vi "Find Steps to Reach End.vi"(0 "Start position":string, 1 "Map":map{string, cluster{string, string}}(c390), 3 "End condition":string, 4 "Instructions":string, 5 "Reach End this many times (1)":u64=1) -> (7 "Steps to reach last end":u64, 8 "End Reached at these steps":u64[](array[numeric]))   [LabVIEW 2020, in "AoC 2023.lvlib"]
uses:
  AoC 2023.lvlib
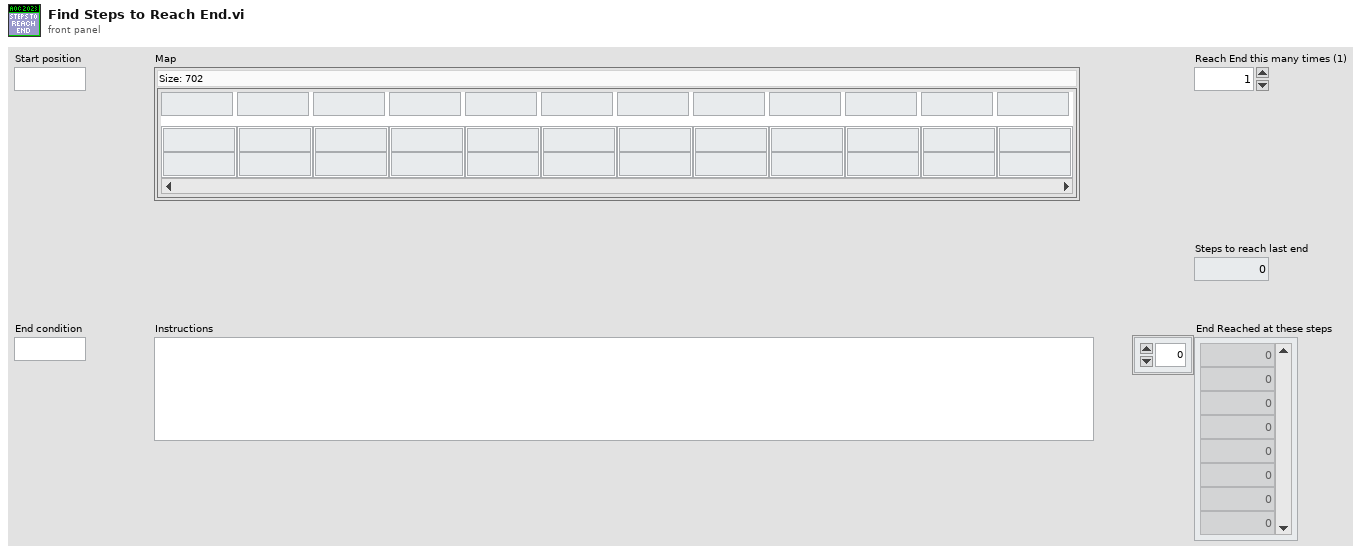
[diagram p1: front panel]
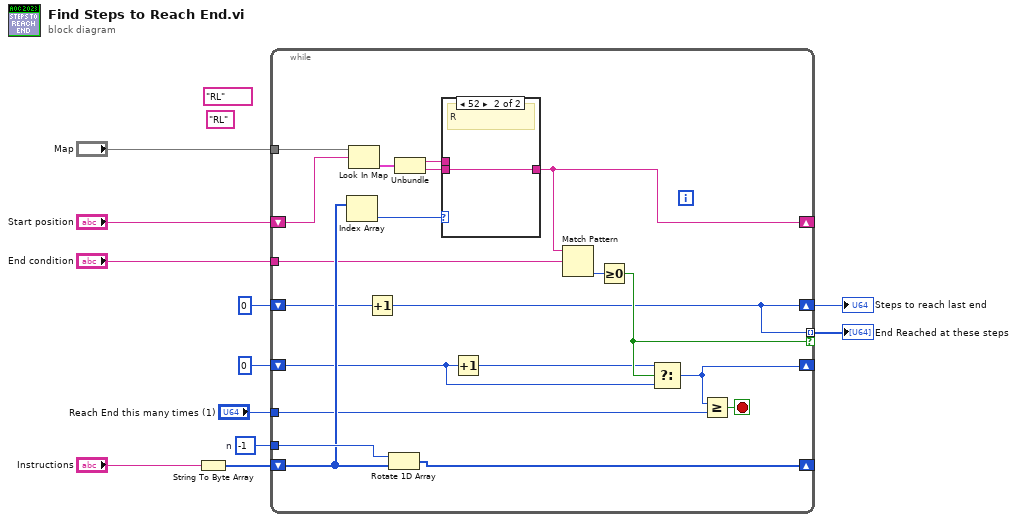
[diagram p0: block diagram]
diagram:
  w7 = -1  # n
  (unwired) "RL"
  (unwired) "RL"
  n1 = String To Byte Array(string="Instructions") -> (unsigned byte array=w6:u8[])
  n2 = while {
    tunnel: "Map" -> [w28]
    shift-right: [w31] -> _
    shift-left: w6 -> [w29]
    shift-right: [w25] -> _
    shift-left: "Start position" -> [w27]
    tunnel: w7 -> [w30]
    shift-right: [w21] -> w9
    shift-left: u64 0 -> [w24]
    tunnel: "End condition" -> [w23]
    tunnel: [w21] -> w1 mode=indexing if=w22
    shift-right: [w17] -> _
    shift-left: u64 0 -> [w20]
    tunnel: "Reach End this many times (1)" -> [w16]
    stop <- w18 stop-if-true
    n3 = Index Array(array=w29) -> (element=w26:u8)  [unwired: 1 in]
    n4 = Look In Map(map=w28, key=w27) -> (value=w15:cluster{string, string})  [unwired: 1 in, 1 out]
    n5 = Increment(x=w24) -> (x+1=w21:u64)
    n6 = Rotate 1D Array(1:w29, 2:w30) -> (0:w31:u8[])
    n7 = Unbundle(w15) -> (w14:string, w13:string)
    n8 = case shown="52" w26 {
      tunnel: w14 -> [w32 _]
      tunnel: w13 -> [_ w33]
      tunnel: [w32 w33] -> w25
      frame 76, Default {
        # "L"
      }
      frame 82 {
        # "R"
      }
    }
    n9 = Increment(x=w20) -> (x+1=w19:u64)
    n10 = Match Pattern(string=w25, regular expression=w23) -> (offset past match=w12:i32)  [unwired: 1 in, 3 out]
    n11 = Greater Or Equal To 0?(x=w12) -> (x >= 0?=w22:bool)
    n12 = Select(t=w19, s=w22, f=w20) -> (s? t:f=w17:u64)
    n13 = Greater Or Equal?(x=w17, y=w16) -> (x >= y?=w18:bool)
  }
  "Steps to reach last end" <- w9
  "End Reached at these steps" <- w1
